vi "FXP_ss_system_matmult.vi"(4 "xk_0_1":T2="xk_0_1_zaxis", 6 "xk_1_0":T2="xk_1_0_zaxis", 7 "ABCD_as_col":T1="ABCD_xaxis", 8 "Uk":fxp<+/-,32,6>, 9 "Ns_nsw":u8=9, 11 "inputValid":bool) -> (0 "Yk":fxp<+/-,36,13>, 2 "finished":bool)   [LabVIEW 2019]
doc: "Multiplies <B>Matrix A</B> by an input <B>Vector b</B>. This operation is useful for FPGA control applications, such as state-feedback control. You can use more than one multiplier to reduce the latency of this operation. To define <B>Matrix A</B>, double-click this Express VI and use the <B>Matrix Data Initialization</B> page to specify a VI, TXT, or CSV file that contains the matrix data. If you do not define <B>Matrix A</B>, this Express VI uses a matrix of zeroes instead.\n--------------------\n\nThis Express VI is configured as follows:\n\n<b>Fixed-Point Configuration</b>\nMatrix A Type: <+/-,32,16>\nVector b Type: <+/-,32,16>\nVector c Type: <+/-,64,36>\nOverflow mode: Truncate [Not Needed]\nRounding mode: Saturate [Not Needed]\n\n<b>Matrix A Configuration</b>\nMatrix Dimensions: 9 * 9\n\n<b>Multiplier Configuration</b>\nNumber of multipliers: 9\nNumber of multiplier pipeline stages: 0\n\n<b>Implementation</b>\nMatrix Vector Multiplication: 11 cycles"
uses:
  fixed-point-ss/typeDefs/x_vec_bram.ctl
  fixed-point-ss/typeDefs/A_as_vec_bram.ctl
  <vilib>/Platform/TimedLoop/XDataNode/timing_clust.ctl
  <vilib>/Platform/TimedLoop/XDataNode/nitl_modes.ctl
  <vilib>/Platform/TimedLoop/XDataNode/wakeup.ctl
  <vilib>/rvi/IPIntegrationNode/IPINode_Typedef/niFpgaIPINodeSupportedFamilies.ctl
  <vilib>/rvi/Emulation/niFpgaSctlEmulationGetInTimedLoop.vi
  <vilib>/Utility/error.llb/Clear Errors.vi
  <vilib>/rvi/DataTransferAndStorage/Container/Common/niFpgaContainerExecOnDevCompGetState.vi
  <vilib>/rvi/Emulation/niFpgaEmulationIsFPGAContextNoSignature.vi
  <vilib>/rvi/DataTransferAndStorage/Container/Common/niFpgaContainerGetUniqueNameForEmu.vi
  <vilib>/rvi/Emulation/niFpgaProcessEmulError.vi
  <vilib>/rvi/errors/nirviReportUnexpectedCaseInternalError (U32).vi
  <vilib>/rvi/Memory/Memory_Emulation/niFpgaMemoryEmulationCacheClearOnFirstRun.vi
  <vilib>/rvi/Memory/Memory_Emulation/nirvimemoryEmulationManagerCache_MakeExclusive.vi
  <vilib>/rvi/Memory/Memory_Emulation/niFpgaMemoryEmulationValidateCache.vi
  <vilib>/rvi/Memory/Memory_Emulation/nirvimemoryEmulationManagerCache_InsertValue.vi
  <vilib>/rvi/Memory/Memory_Emulation/nirvimemoryEmulationManagerCache_ReleaseExclusive.vi
  <vilib>/rvi/Memory/Memory_Emulation/nirvimemoryEmulationManagerCache_GetValue.vi
  <vilib>/rvi/Memory/Memory_Emulation/nirvimemoryEmulationManagerCache_SetValue.vi
  <vilib>/rvi/Emulation/niFpgaSctlEmulationResourceMgr.vi
  <vilib>/rvi/IPIntegrationNode/IPINode_Utilities/niFpgaIPINodeSimCore.vi
  <vilib>/Platform/TimedLoop/XDataNode/XDataNode.xnode
  <vilib>/rvi/DataTransferAndStorage/Container/XNode/niFpgaContainer.xnode
  <vilib>/rvi/Memory/Memory_Emulation/niFpgaMemoryEmulationRefIn.vi
  <vilib>/rvi/XilinxIP/XIPIN_XNode/niFpgaXIPIN.xnode
  MAC01/MAC01_2_75F243352369479695E2AED5F4206BF1.dll
  <vilib>/rvi/IPIntegrationNode/IPINode_Xnode/niFpgaIPINode.xnode
  <vilib>/Platform/TimedLoop/XDataNode/XDNodeRunTimeDep.lvlib
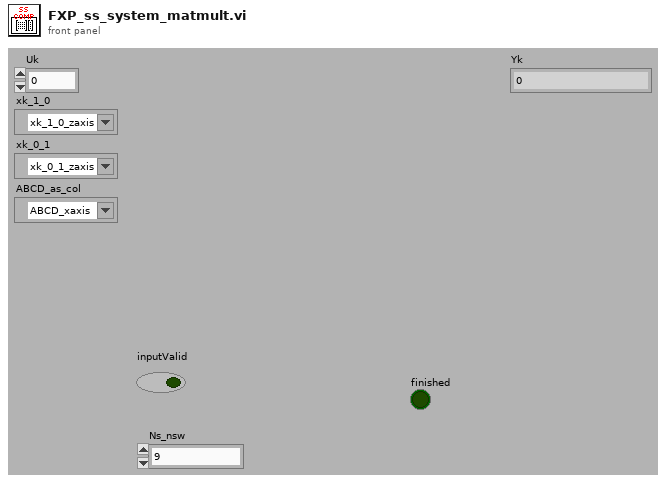
[diagram p1: front panel]
types:
  T1 = typedef "A_as_vec_bram.ctl" = refnum<k21>
  T2 = typedef "x_vec_bram.ctl" = refnum<k21>
  T3 = typedef "niFpgaIPINodeSupportedFamilies.ctl" = cluster{"unlimited?":bool, "supported targets":string[]}
  T4 = typedef "XDNodeRunTimeDep.lvlib/timing_clust.ctl" = cluster{"Expected End [f-1]":u64, "Actual End [f-1]":u64, "Finished Late? [f-1]":bool, "Expected End [i-1]":u64, "Actual End [i-1]":u64, "Finished Late? [i-1]":bool, "Expected Start [i]":u64, "Actual Start [i]":u64, "Expected Start [f]":u64, "Actual Start [f]":u64, "Source Name":string, "Structure Name":string, "Period":i64, "Deadline":i64, "Offset":i64, "Start":i64, "Priority":i32, "Timeout":i32, "Mode":T5, "Wakeup Reason":T6, "Error":errorcluster, "Source Type":string, "Secondary Source Type":string, "Global End Time":u64, "Global Start Time":u64, "Frame Duration":u64, "Iteration Duration":u64, "Assigned CPU":i32, "I/O Scan Engine Mode":u32}
  T5 = typedef "XDNodeRunTimeDep.lvlib/nitl_modes.ctl" = enum32{"No Change", "Process missed periods, maintain original phase", "Discard missed periods, maintain original phase", "Process missed periods, ignore original phase", "Discard missed periods, ignore original phase"}
  T6 = typedef "XDNodeRunTimeDep.lvlib/wakeup.ctl" = enum32{"Normal", "Aborted", "Asynchronous wakeup", "Timing source error", "Timed loop error", "Timeout"}
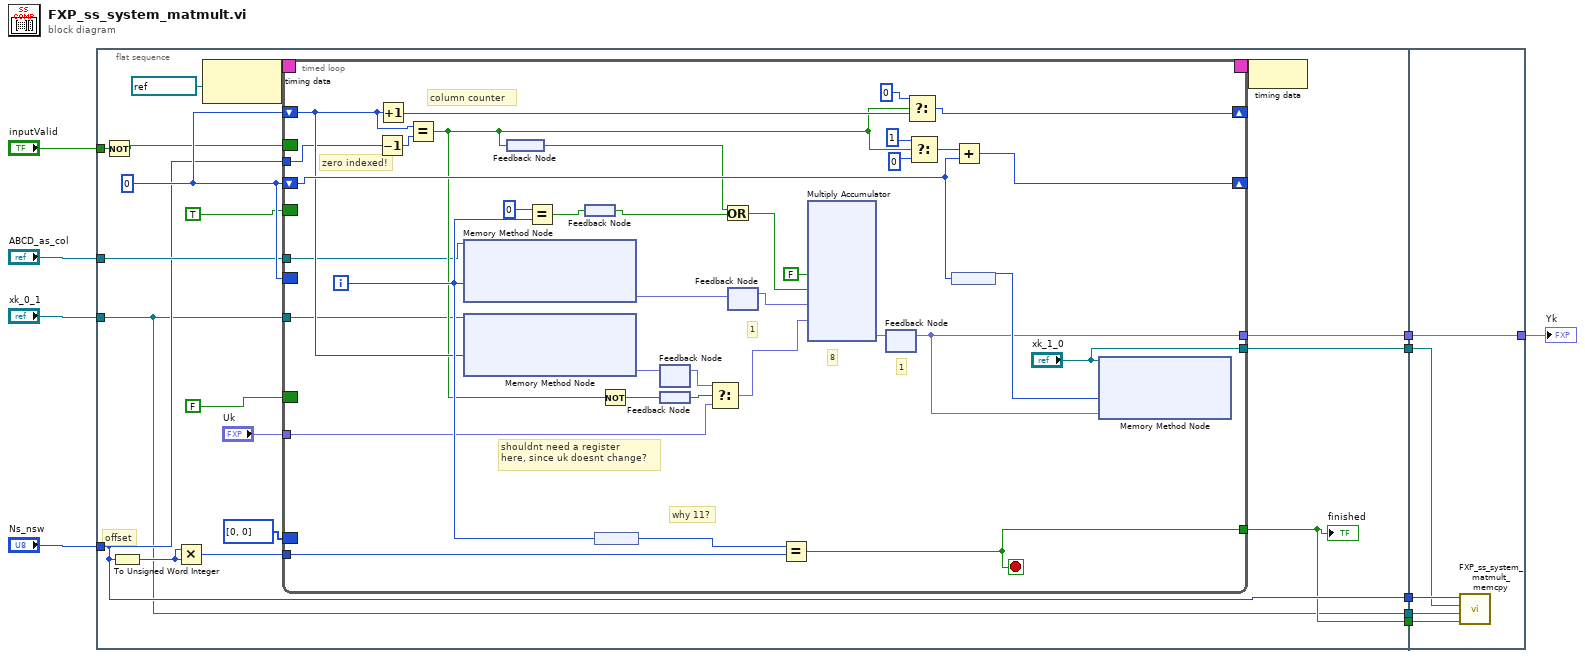
[diagram p0: block diagram]
diagram:
  n1 = flat-sequence {
    tunnel: [w17] -> w10
    tunnel: "xk_0_1" -> [w11]
    tunnel: "ABCD_as_col" -> [w16]
    tunnel: "Ns_nsw" -> [w14]
    tunnel: "inputValid" -> [w15]
    tunnel: [w14] -> w4
    tunnel: [w13] -> w3
    tunnel: [w12] -> w2
    tunnel: [w11] -> w1
    tunnel: w10 -> [w135]
    tunnel: [w135] -> w9
    tunnel: w4 -> [w134]
    tunnel: w3 -> [w133]
    tunnel: w2 -> [w132]
    tunnel: w1 -> [w131]
    frame #0 {
      w26 = u8 0
      # "offset"
      n2 = Not(x=w15) -> (.not. x?=w24:bool)
      n3 = To Unsigned Word Integer(number=w14) -> (unsigned 16bit integer=w25:u16)
      n4 = Multiply(x=w25, y=w25) -> (x*y=w22:u16)
      n5 = node-c288(refnum<k21> "80MHz" ("Source Name")) -> (w28:T4)
      n6 = timed-loop {
        timing: w28 -> [_]
        timing-out: [_] -> w27
        shift-right: [w60] -> _
        shift-left: w26 -> [w57]
        shift-right: [w64] -> _
        shift-left: w26 -> [w49]
        border: w24 -> [_]
        border: w26 -> [_]
        tunnel: w22 -> [w50]
        border: TRUE -> [_]
        border: i32[] [0, 0] -> [_]
        tunnel: "Uk" -> [w42]
        tunnel: [w41] -> w13
        border: FALSE -> [_]
        tunnel: [w33] -> w17
        tunnel: w11 -> [w32]
        tunnel: w16 -> [w31]
        tunnel: w14 -> [w30]
        tunnel: ["xk_1_0"] -> w12
        i -> [w52]
        stop <- w41 stop-if-true
        # "8"
        # "shouldnt need a register\nhere, since uk doesnt change?"
        # "why 11?"
        # "1"
        # "1"
        # "zero indexed!"
        # "column counter"
        n7 = Decrement(x=w30) -> (x-1=w56:u8)
        n8 = Increment(x=w49) -> (x+1=w59:u8)
        n9 = Equal?(x=w49, y=w56) -> (x = y?=w43:bool)
        n10 = xnode ("Memory Method Node")("Address"=w52, "Memory In"=w31) -> ("Data"=w46:fxp<+/-,32,7>)  [unwired: 1 out]
        n11 = xnode ("Memory Method Node")("Address"=w49, "Memory In"=w32) -> ("Data"=w40:fxp<+/-,32,6>)  [unwired: 1 out]
        n12 = feedback #1() -> (w55:bool)
        n13 = feedback-in #1(w43) -> ()
        n14 = Equal?(x=0, y=w52) -> (x = y?=w47:bool)
        n15 = feedback #2() -> (w48:bool)
        n16 = feedback-in #2(w47) -> ()
        n17 = feedback #3() -> (w53:i32)
        n18 = feedback-in #3(w52) -> ()
        n19 = Not(x=w43) -> (.not. x?=w34:bool)
        n20 = feedback #4() -> (w39:fxp<+/-,32,6>)  [unwired: 1 in]
        n21 = feedback-in #4(w40) -> ()
        n22 = feedback #5() -> (w35:bool)
        n23 = feedback-in #5(w34) -> ()
        n24 = Select(t=w39, s=w35, f=w42) -> (s? t:f=w36:fxp<+/-,32,6>)
        n25 = Or(x=w55, y=w48) -> (x .or. y?=w37:bool)
        n26 = feedback-in #6(w46) -> ()
        n27 = feedback #6() -> (w38:fxp<+/-,32,7>)  [unwired: 1 in]
        n28 = Equal?(x=w53, y=w50) -> (x = y?=w41:bool)
        n29 = xnode ("Multiply Accumulator")("sclr"=FALSE, "bypass"=w37, "a"=w38, "b"=w36) -> ("s"=w45:fxp<+/-,36,13>)  [unwired: 1 in]
        n30 = feedback #7() -> (w33:fxp<+/-,36,13>)  [unwired: 1 in]
        n31 = feedback-in #7(w45) -> ()
        n32 = Select(t=u8 0, s=w43, f=w59) -> (s? t:f=w64:u8)
        n33 = Select(t=u8 1, s=w43, f=u8 0) -> (s? t:f=w61:u8)
        n34 = feedback #8() -> (w44:u8)
        n35 = feedback-in #8(w57) -> ()
        n36 = Add(x=w61, y=w57) -> (x+y=w60:u8)
        n37 = xnode ("Memory Method Node")("Address"=w44, "Data"=w33, "Memory In"="xk_1_0") -> ()  [unwired: 1 out]
      }
      "finished" <- w13
      n38 = node-c288(w27) -> ()
    }
    frame #1 {
      n39 = call "FXP_ss_system_matmult_memcpy.vi"("InputValid"=w133, "xk_0_1"=w131, "xk_1_0"=w132, "Ns_nsw"=w134) -> ()  [unwired: 8 in]
    }
  }
  "Yk" <- w9
